vi "STS Cluster to REG.vi"(0 "STS REG":T1) -> (4 "U16":u16)   [LabVIEW 2019, in "ModbusSp.lvclass"]
uses:
  ModbusSp.lvclass
  STS REG.ctl
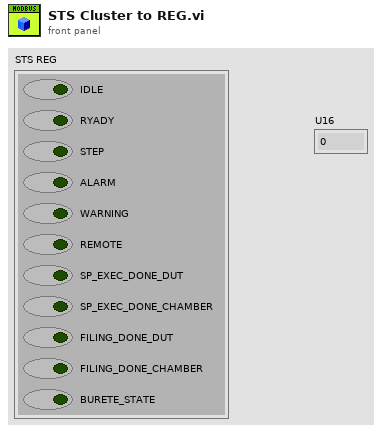
[diagram p1: front panel]
types:
  T1 = typedef "STS REG.ctl" = cluster{"IDLE":bool, "RYADY":bool, "STEP":bool, "ALARM":bool, "WARNING":bool, "REMOTE":bool, "SP_EXEC_DONE_DUT":bool, "SP_EXEC_DONE_CHAMBER":bool, "FILING_DONE_DUT":bool, "FILING_DONE_CHAMBER":bool, "BURETE_STATE":bool}
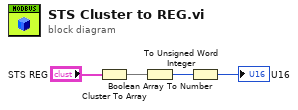
[diagram p0: block diagram]
diagram:
  n1 = Cluster To Array(cluster="STS REG") -> (array=w3:bool[])
  n2 = Boolean Array To Number(Boolean array=w3) -> (number=w2:u32)
  n3 = To Unsigned Word Integer(number=w2) -> (unsigned 16bit integer=→"U16":u16)
